vi "storeADCMixedToArray-wang-test2not simplified2.vi"(0 "String":string) -> (18 "Graph Data":T1)   [LabVIEW 2014]
uses:
  main/controls/Graph Data.ctl
  <vilib>/Utility/miscctls.llb/LVAnnotationListTypeDef.ctl
  <vilib>/Utility/miscctls.llb/LVCursorListTypeDef.ctl
  main/global/Global ADCarray.vi
panel:
  out "Array - String":string[](array[string])
  out "Array - Numeric":u8[](array[numeric])
  out "Waveform":waveform(dbl)
  out "Graph":waveform(i32)[](graph)
  out "Numeric 2":i32
  out "Numeric":i32
  out "CH7":i32[](array[numeric])
  out "CH6":i32[](array[numeric])
  out "CH5":i32[](array[numeric])
  out "CH4":i32[](array[numeric])
  out "CH3":i32[](array[numeric])
  out "CH2":i32[](array[numeric])
  out "CH1":i32[](array[numeric])
  out "CH0":i32[](array[numeric])
  out "TotalTrigger":i32
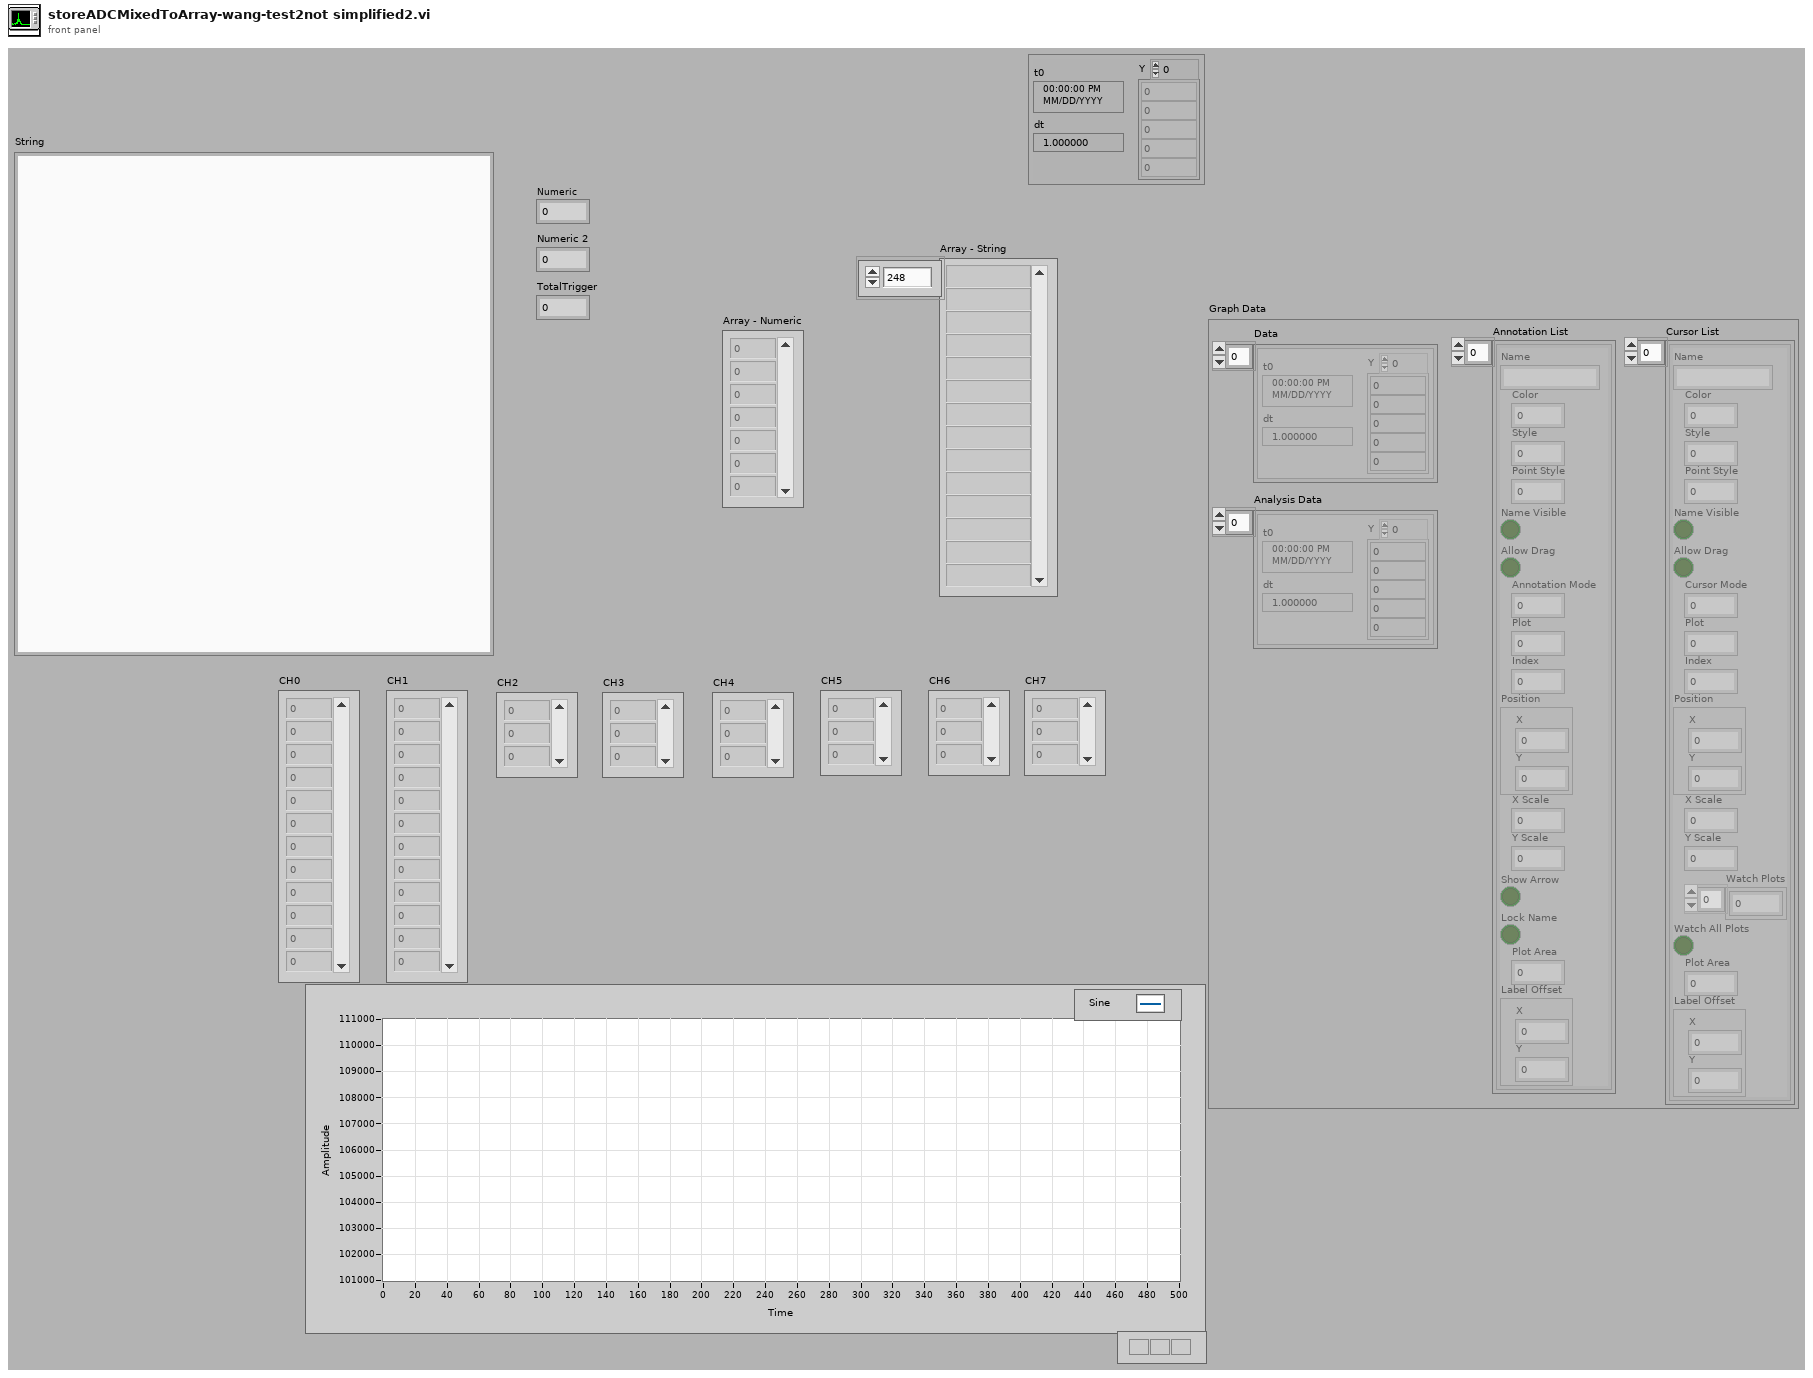
[diagram p1: front panel]
types:
  T1 = typedef "Graph Data.ctl" = cluster{"Data":waveform(dbl)[], "Annotation List":T2, "Cursor List":T3, "Analysis Data":waveform(dbl)[]}
  T2 = typedef "LVAnnotationListTypeDef.ctl" = cluster{"Name":string, "Color":u32, "Style":u8, "Point Style":u8, "Name Visible":bool, "Allow Drag":bool, "Annotation Mode":u32, "Plot":i32, "Index":i32, "Position":cluster{"X":dbl, "Y":dbl}, "X Scale":u32, "Y Scale":u32, "Show Arrow":bool, "Lock Name":bool, "Plot Area":i32, "Label Offset":cluster{"X":dbl, "Y":dbl}}[]
  T3 = typedef "LVCursorListTypeDef.ctl" = cluster{"Name":string, "Color":u32, "Style":u8, "Point Style":u8, "Name Visible":bool, "Allow Drag":bool, "Cursor Mode":u32, "Plot":i32, "Index":i32, "Position":cluster{"X":dbl, "Y":dbl}, "X Scale":u32, "Y Scale":u32, "Watch Plots":i32[], "Watch All Plots":bool, "Plot Area":i32, "Label Offset":cluster{"X":dbl, "Y":dbl}}[]
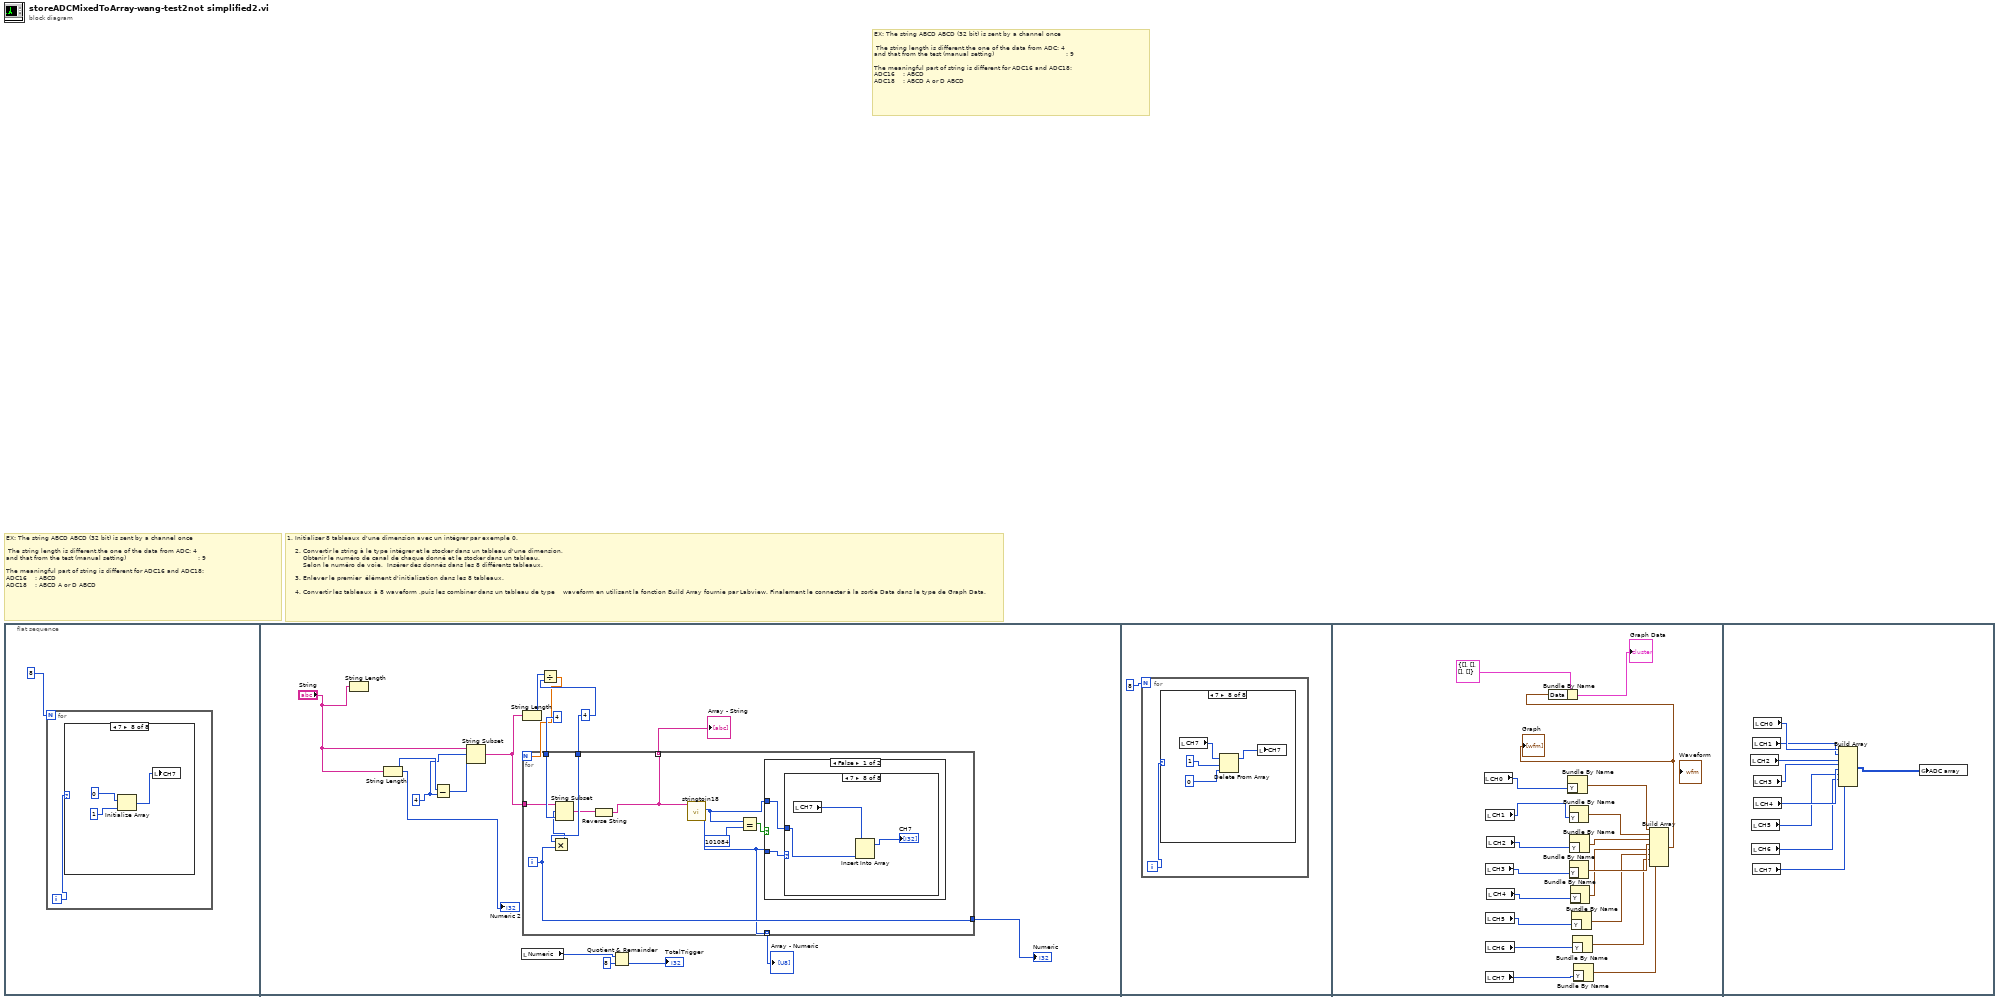
[diagram p0: block diagram]
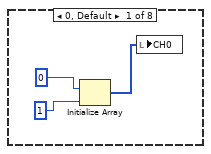
[diagram p2: hidden frame]
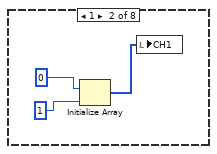
[diagram p3: hidden frame]
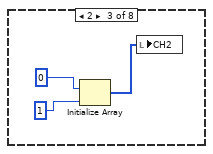
[diagram p4: hidden frame]
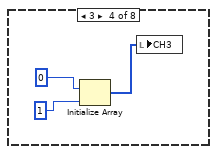
[diagram p5: hidden frame]
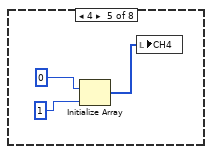
[diagram p6: hidden frame]
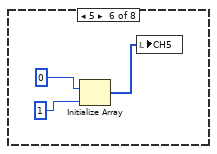
[diagram p7: hidden frame]
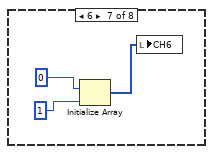
[diagram p8: hidden frame]
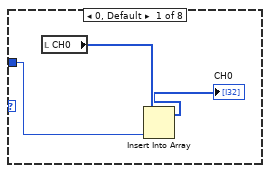
[diagram p9: hidden frame]
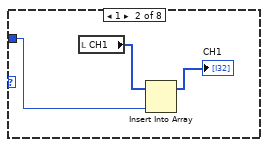
[diagram p10: hidden frame]
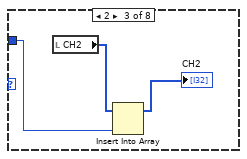
[diagram p11: hidden frame]
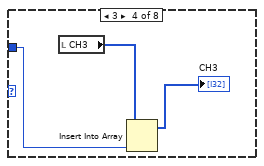
[diagram p12: hidden frame]
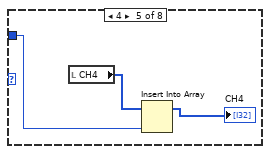
[diagram p13: hidden frame]
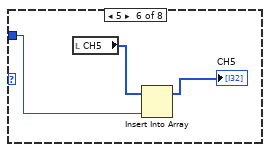
[diagram p14: hidden frame]
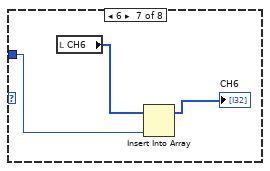
[diagram p15: hidden frame]
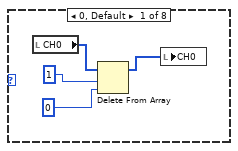
[diagram p17: hidden frame]
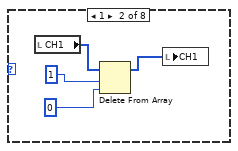
[diagram p18: hidden frame]
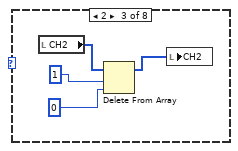
[diagram p19: hidden frame]
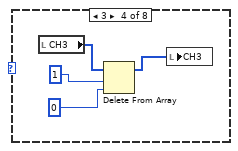
[diagram p20: hidden frame]
diagram:
  # "1. Initialiser 8 tableaux d'une dimension avec un intégrer par exemple 0.\n\n    2.\tConvertir le string à le type intégrer et le stocker dans un tableau d'une dimension,\n        Obtenir le numéro de canal de chaque donné et le stocker dans un tableau.  \n        Selon le numéro de voie,  Insérer des donnés dans les 8 différents tableaux.\n\n    3. Enlever le premier  élément d'initialisation dans les 8 tableaux.\n\n    4. Convertir les tableaux à 8 waveform ,puis les combiner dans un tableau de type    waveform en utilisant la fonction Build Array fournie par Labview. Finalement le connecter à la sortie Data dans le type de Graph Data."
  # "EX: The string ABCD ABCD (32 bit) is sent by a channel once                \n\n The string length is different,the one of the data from ADC: 4\nand that from the test (manual setting)                                    : 9\n\nThe meaningful part of string is different for ADC16 and ADC18:\nADC16    : ABCD                          \nADC18    : ABCD A or D ABCD"
  # "EX: The string ABCD ABCD (32 bit) is sent by a channel once                \n\n The string length is different,the one of the data from ADC: 4\nand that from the test (manual setting)                                    : 9\n\nThe meaningful part of string is different for ADC16 and ADC18:\nADC16    : ABCD                          \nADC18    : ABCD A or D ABCD"
  n1 = flat-sequence {
    frame #0 {
      n2 = for {
        N: 8 -> [_]
        i -> [w2]
        n3 = case shown="7" w2 {
          frame 0, Default {
            n4 = Initialize Array(0, 1) -> (w3:i32[])
            n5 = local write "CH0"(w3) -> ()
          }
          frame 1 {
            n6 = Initialize Array(0, 1) -> (w6:i32[])
            n7 = local write "CH1"(w6) -> ()
          }
          frame 2 {
            n8 = Initialize Array(0, 1) -> (w9:i32[])
            n9 = local write "CH2"(w9) -> ()
          }
          frame 3 {
            n10 = Initialize Array(0, 1) -> (w12:i32[])
            n11 = local write "CH3"(w12) -> ()
          }
          frame 4 {
            n12 = Initialize Array(0, 1) -> (w15:i32[])
            n13 = local write "CH4"(w15) -> ()
          }
          frame 5 {
            n14 = Initialize Array(0, 1) -> (w18:i32[])
            n15 = local write "CH5"(w18) -> ()
          }
          frame 6 {
            n16 = Initialize Array(0, 1) -> (w21:i32[])
            n17 = local write "CH6"(w21) -> ()
          }
          frame 7 {
            n18 = Initialize Array(0, 1) -> (w24:i32[])
            n19 = local write "CH7"(w24) -> ()
          }
        }
      }
    }
    frame #1 {
      w35 = 4
      w38 = 4
      n20 = String Length(string="String") -> ()  [unwired: 1 out]
      n21 = String Length(string="String") -> (length=w41:i32)
      "Numeric 2" <- w41
      n22 = Subtract(x=w41, y=w38) -> (x-y=w39:i32)
      n23 = String Subset(string="String", offset (0)=w38, length (rest)=w39) -> (substring=w33:string)
      n24 = local read "Numeric"() -> (w30:i32)
      n25 = String Length(string=w33) -> (length=w36:i32)
      n26 = Divide(x=w36, y=w35) -> (x/y=w34:dbl)
      n27 = for {
        N: w34 -> [_]
        tunnel: 4 -> [w52]
        tunnel: w35 -> [w51]
        tunnel: [w47] -> w40
        tunnel: w33 -> [w48]
        tunnel: [w46] -> w28 mode=indexing
        tunnel: [w45] -> w27 mode=indexing
        i -> [w47]
        n28 = Multiply(x=w51, y=w47) -> (x*y=w50:i32)
        n29 = String Subset(string=w48, offset (0)=w50, length (rest)=w52) -> (substring=w49:string)
        n30 = Reverse String(1:w49) -> (0:w45:string)
        n31 = call "stringtoin18.vi"("input_string"=w45) -> ("channel"=w46:u8, "outputComplemented_int"=w42:i32)  [unwired: 7 in, 2 out]
        n32 = Equal?(x=w42, y=101084) -> (x = y?=w43:bool)
        n33 = case shown="False" w43 {
          tunnel: w42 -> [w54 _]
          tunnel: w46 -> [w53 _]
          frame False {
            n34 = case shown="7" w53 {
              tunnel: w54 -> [w55 w58 w61 w64 w67 w70 w73 w76]
              frame 0, Default {
                n35 = local read "CH0"() -> (w57:i32[])
                n36 = Insert Into Array(array=w57, new element=w55) -> (→"CH0":i32[])  [unwired: 1 in]
              }
              frame 1 {
                n37 = local read "CH1"() -> (w60:i32[])
                n38 = Insert Into Array(array=w60, new element=w58) -> (→"CH1":i32[])  [unwired: 1 in]
              }
              frame 2 {
                n39 = local read "CH2"() -> (w63:i32[])
                n40 = Insert Into Array(array=w63, new element=w61) -> (→"CH2":i32[])  [unwired: 1 in]
              }
              frame 3 {
                n41 = local read "CH3"() -> (w66:i32[])
                n42 = Insert Into Array(array=w66, new element=w64) -> (→"CH3":i32[])  [unwired: 1 in]
              }
              frame 4 {
                n43 = local read "CH4"() -> (w69:i32[])
                n44 = Insert Into Array(array=w69, new element=w67) -> (→"CH4":i32[])  [unwired: 1 in]
              }
              frame 5 {
                n45 = local read "CH5"() -> (w72:i32[])
                n46 = Insert Into Array(array=w72, new element=w70) -> (→"CH5":i32[])  [unwired: 1 in]
              }
              frame 6 {
                n47 = local read "CH6"() -> (w75:i32[])
                n48 = Insert Into Array(array=w75, new element=w73) -> (→"CH6":i32[])  [unwired: 1 in]
              }
              frame 7 {
                n49 = local read "CH7"() -> (w77:i32[])
                n50 = Insert Into Array(array=w77, new element=w76) -> (→"CH7":i32[])  [unwired: 1 in]
              }
            }
          }
          frame True {
          }
        }
      }
      "Numeric" <- w40
      "Array - Numeric" <- w28
      "Array - String" <- w27
      n51 = Quotient & Remainder(x=w30, y=8) -> (floor(x/y)=→"TotalTrigger":i32)  [unwired: 1 out]
    }
    frame #2 {
      n52 = for {
        N: 8 -> [_]
        i -> [w80]
        n53 = case shown="7" w80 {
          frame 0, Default {
            n54 = local read "CH0"() -> (w84:i32[])
            n55 = Delete From Array(array=w84, length=1, index=0) -> (array with subset deleted=w81:i32[])  [unwired: 1 out]
            n56 = local write "CH0"(w81) -> ()
          }
          frame 1 {
            n57 = local read "CH1"() -> (w88:i32[])
            n58 = Delete From Array(array=w88, length=1, index=0) -> (array with subset deleted=w85:i32[])  [unwired: 1 out]
            n59 = local write "CH1"(w85) -> ()
          }
          frame 2 {
            n60 = local read "CH2"() -> (w92:i32[])
            n61 = Delete From Array(array=w92, length=1, index=0) -> (array with subset deleted=w89:i32[])  [unwired: 1 out]
            n62 = local write "CH2"(w89) -> ()
          }
          frame 3 {
            n63 = local read "CH3"() -> (w96:i32[])
            n64 = Delete From Array(array=w96, length=1, index=0) -> (array with subset deleted=w93:i32[])  [unwired: 1 out]
            n65 = local write "CH3"(w93) -> ()
          }
          frame 4 {
            n66 = local read "CH4"() -> (w100:i32[])
            n67 = Delete From Array(array=w100, length=1, index=0) -> (array with subset deleted=w97:i32[])  [unwired: 1 out]
            n68 = local write "CH4"(w97) -> ()
          }
          frame 5 {
            n69 = local read "CH5"() -> (w104:i32[])
            n70 = Delete From Array(array=w104, length=1, index=0) -> (array with subset deleted=w101:i32[])  [unwired: 1 out]
            n71 = local write "CH5"(w101) -> ()
          }
          frame 6 {
            n72 = local read "CH6"() -> (w108:i32[])
            n73 = Delete From Array(array=w108, length=1, index=0) -> (array with subset deleted=w105:i32[])  [unwired: 1 out]
            n74 = local write "CH6"(w105) -> ()
          }
          frame 7 {
            n75 = local read "CH7"() -> (w112:i32[])
            n76 = Delete From Array(array=w112, length=1, index=0) -> (array with subset deleted=w109:i32[])  [unwired: 1 out]
            n77 = local write "CH7"(w109) -> ()
          }
        }
      }
    }
    frame #3 {
      n78 = local read "CH0"() -> (w131:i32[])
      n79 = local read "CH3"() -> (w123:i32[])
      n80 = local read "CH7"() -> (w127:i32[])
      n81 = local read "CH1"() -> (w129:i32[])
      n82 = local read "CH5"() -> (w125:i32[])
      n83 = local read "CH6"() -> (w126:i32[])
      n84 = local read "CH2"() -> (w122:i32[])
      n85 = local read "CH4"() -> (w124:i32[])
      n86 = Bundle By Name("Y"=w131) -> (w130:waveform(i32))  [unwired: 1 in]
      n87 = Bundle By Name("Y"=w129) -> (w128:waveform(i32))  [unwired: 1 in]
      n88 = Bundle By Name("Y"=w123) -> (w120:waveform(i32))  [unwired: 1 in]
      n89 = Bundle By Name("Y"=w122) -> (w121:waveform(i32))  [unwired: 1 in]
      n90 = Bundle By Name("Y"=w124) -> (w116:waveform(i32))  [unwired: 1 in]
      n91 = Bundle By Name("Y"=w125) -> (w119:waveform(i32))  [unwired: 1 in]
      n92 = Bundle By Name("Y"=w126) -> (w118:waveform(i32))  [unwired: 1 in]
      n93 = Bundle By Name("Y"=w127) -> (w117:waveform(i32))  [unwired: 1 in]
      n94 = Build Array(w130, w128, w121, w120, w116, w119, w118, w117) -> (w115:waveform(i32)[])
      "Graph" <- w115
      n95 = Bundle By Name(cluster=T1 {"Data"=[], "Annotation List"=[], "Cursor List"=[], "Analysis Data"=[]} ("Graph Data"), "Data"=w115) -> (→"Graph Data":T1)
    }
    frame #4 {
      n96 = local read "CH2"() -> (w138:i32[])
      n97 = local read "CH5"() -> (w135:i32[])
      n98 = local read "CH6"() -> (w134:i32[])
      n99 = local read "CH1"() -> (w139:i32[])
      n100 = local read "CH7"() -> (w133:i32[])
      n101 = local read "CH3"() -> (w137:i32[])
      n102 = local read "CH0"() -> (w140:i32[])
      n103 = local read "CH4"() -> (w136:i32[])
      n104 = Build Array(w140, w139, w138, w137, w136, w135, w134, w133) -> (w132:i32[][])
      n105 = global write "Global ADCarray.vi" "ADC array"(w132) -> ()
    }
  }
